vi "Configure Channel.vi"(0 "VISA resource name":refnum<visa-resource-name>, 1 "Vertical Range (0.04)":dbl=0.04 format="%.3e", 2 "Channel Polarity (Normal)":i32(ring) items=["Normal", "Inverted"], 3 "Vertical Coupling (DC 1 MOhm)":i32(ring)=2 items=["AC", "DC 50 Ohm", "DC 1 MOhm", "AC 1 MOhm", "Ground"], 5 "Channel (1)":i32(ring)=1 items=["1"=1, "2"=2, "3"=3, "4"=4, "External"=5], 9 "Channel Enabled (T: On)":bool=TRUE, 11 "error in (no error)":errorcluster, 12 "Vertical Offset (0.0)":dbl format="%^.3e", 13 "Channel Skew (0.0)":dbl format="%^.3e") -> (4 "VISA resource name out":refnum<visa-resource-name>, 15 "error out":errorcluster)   [LabVIEW 2020, in "Rohde&Schwarz RTx Oscilloscopes.lvlib"]
doc: "This VI configures the common attributes of the oscilloscope's channel subsystem for a particular channel. These attributes are the vertical range, vertical offset, coupling, probe attenuation, and channel enabled.\n\nAttributes:\nRSRTX_ATTR_CHANNEL_ENABLED\nRSRTX_ATTR_VERTICAL_RANGE\nRSRTX_ATTR_CHANNEL_OFFSET\nRSRTX_ATTR_VERTICAL_COUPLING\nRSRTX_ATTR_CHANNEL_POLARITY\nRSRTX_ATTR_CHANNEL_SKEW\n\nRemote-control commands:\nCHANnel<m>:STATe\nCHANnel<m>:RANGe\nCHANnel<m>:OFFSet\nCHANnel<m>:COUPling\nCHANnel<m>:POLarity\nCHANnel<m>:SKEW"
uses:
  Rohde&Schwarz RTx Oscilloscopes.lvlib
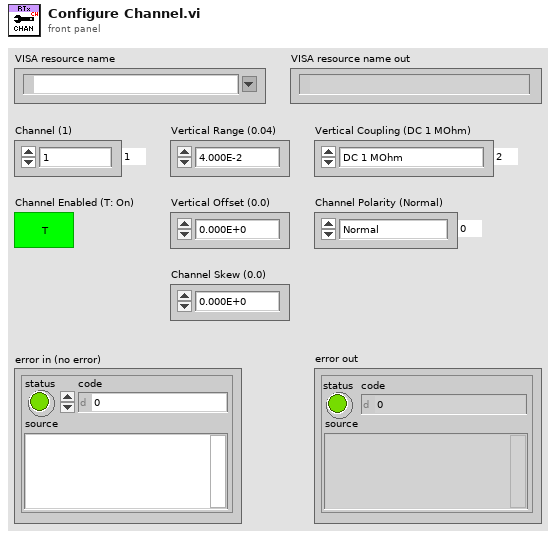
[diagram p1: front panel]
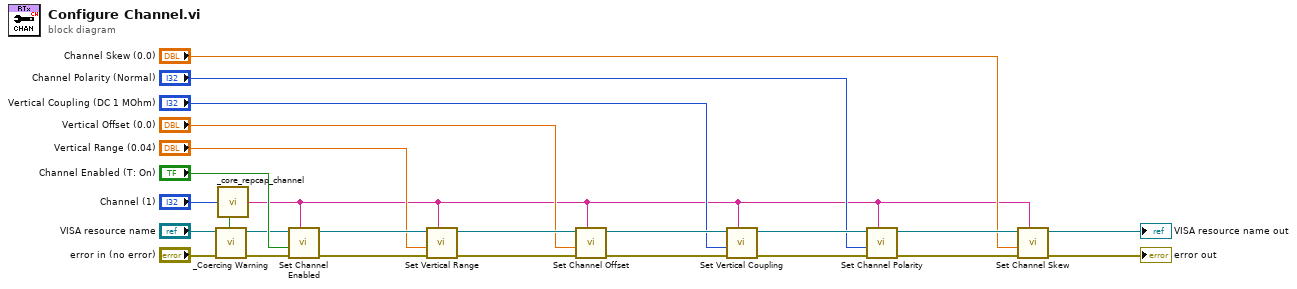
[diagram p0: block diagram]
diagram:
  n1 = call "_core_repcap_channel.vi"("Channel In"="Channel (1)") -> ("In Range?"=w2:bool, "Channel Identifier Out"=w1:string)  [unwired: 1 out]
  n2 = call "_Coercing Warning.vi"("In Range?"=w2, "error in"="error in (no error)", "VISA resource name"="VISA resource name") -> ("error out"=w3:errorcluster, "VISA resource name out"=w5:refnum<visa-resource-name>)  [unwired: 7 in]
  n3 = call "Set Channel Enabled"("Repeated Capabilities"=w1, "error in (no error)"=w3, "Channel Enabled (OFF)"="Channel Enabled (T: On)", "instrument handle"=w5) -> ("error out"=w19:errorcluster, "instrument handle out"=w24:refnum<visa-resource-name>)  [unwired: 6 in]
  n4 = call "Set Vertical Range"("Repeated Capabilities"=w1, "error in (no error)"=w19, "Vertical Range (0.0)"="Vertical Range (0.04)", "instrument handle"=w24) -> ("error out"=w20:errorcluster, "instrument handle out"=w23:refnum<visa-resource-name>)  [unwired: 6 in]
  n5 = call "Set Channel Offset"("Repeated Capabilities"=w1, "error in (no error)"=w20, "Channel Offset (0.0)"="Vertical Offset (0.0)", "instrument handle"=w23) -> ("error out"=w21:errorcluster, "instrument handle out"=w22:refnum<visa-resource-name>)  [unwired: 6 in]
  n6 = call "Set Vertical Coupling"("Repeated Capabilities"=w1, "error in (no error)"=w21, "Vertical Coupling (0 - AC)"="Vertical Coupling (DC 1 MOhm)", "instrument handle"=w22) -> ("error out"=w16:errorcluster, "instrument handle out"=w15:refnum<visa-resource-name>)  [unwired: 6 in]
  n7 = call "Set Channel Polarity"("Repeated Capabilities"=w1, "error in (no error)"=w16, "Channel Polarity (0 - Normal)"="Channel Polarity (Normal)", "instrument handle"=w15) -> ("error out"=w18:errorcluster, "instrument handle out"=w17:refnum<visa-resource-name>)  [unwired: 6 in]
  n8 = call "Set Channel Skew"("Repeated Capabilities"=w1, "error in (no error)"=w18, "Channel Skew (0.0)"="Channel Skew (0.0)", "instrument handle"=w17) -> ("error out"=→"error out":errorcluster, "instrument handle out"=→"VISA resource name out":refnum<visa-resource-name>)  [unwired: 6 in]
